vi "MessageReceiver_NewParse.vi"(0 "STOMP In":refnum<class "STOMP.lvclass">, 5 "error in (no error)":errorcluster) -> (14 "STOMP out":refnum<class "STOMP.lvclass">, 19 "error out":errorcluster)   [LabVIEW 2017, in "LabVIEW STOMP.lvlib" / "STOMP.lvclass"]
uses:
  STOMP.lvclass
  Typedefs/Type_MessageParserState.ctl
  Typedefs/Type_ServerFrame.ctl
  Typedefs/Type_ServerFrameType.ctl
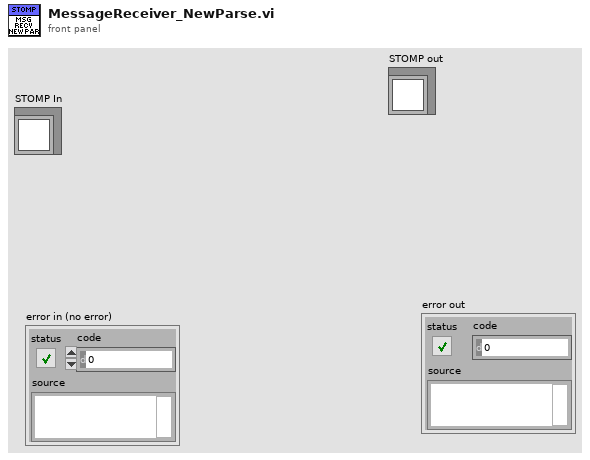
[diagram p1: front panel]
types:
  T1 = typedef "LabVIEW STOMP.lvlib/STOMP.lvclass/Type_ServerFrame.ctl" = cluster{"Type":T2, "Headers":cluster{"Header":string, "Value":string}[], "Body":string}
  T2 = typedef "LabVIEW STOMP.lvlib/STOMP.lvclass/Type_ServerFrameType.ctl" = enum16{"Undefined", "MESSAGE", "CONNECTED", "RECEIPT", "ERROR"}
  T3 = typedef "LabVIEW STOMP.lvlib/STOMP.lvclass/Type_MessageParserState.ctl" = enum16{"WaitForFrame", "ReadCommand", "ReadHeaders", "ReadBody", "FrameReady"}
  T4 = enum16{"Standard", "Buffered", "CRLF", "Immediate"}
  T5 = typedef "STOMP Connection Manager.lvclass/ObjectAttributes.ctl" = cluster{"address":string, "port":u16, "ConnectionRef":refnum<k5>, "messageQueue":refnum<queue>, "receiptQueue":refnum<queue>, "errorQueue":refnum<queue>, "sendQueue":refnum<queue>, "currentReceiptNumber":u64, "currentSubscriptionId":u64, "closeConnection":bool, "activeSubscriptions":T6[]}
  T6 = typedef "LabVIEW STOMP.lvlib/STOMP.lvclass/Type_ActiveSubscription.ctl" = cluster{"id":u64, "receipt":bool, "Destination":string, "ack":T7, "headers":T8[]}
  T7 = typedef "LabVIEW STOMP.lvlib/STOMP.lvclass/Type_AckHeader.ctl" = enum16{"auto", "client", "client-individual"}
  T8 = typedef "LabVIEW STOMP.lvlib/STOMP.lvclass/Type_FrameHeader.ctl" = cluster{"Header":string, "Value":string}
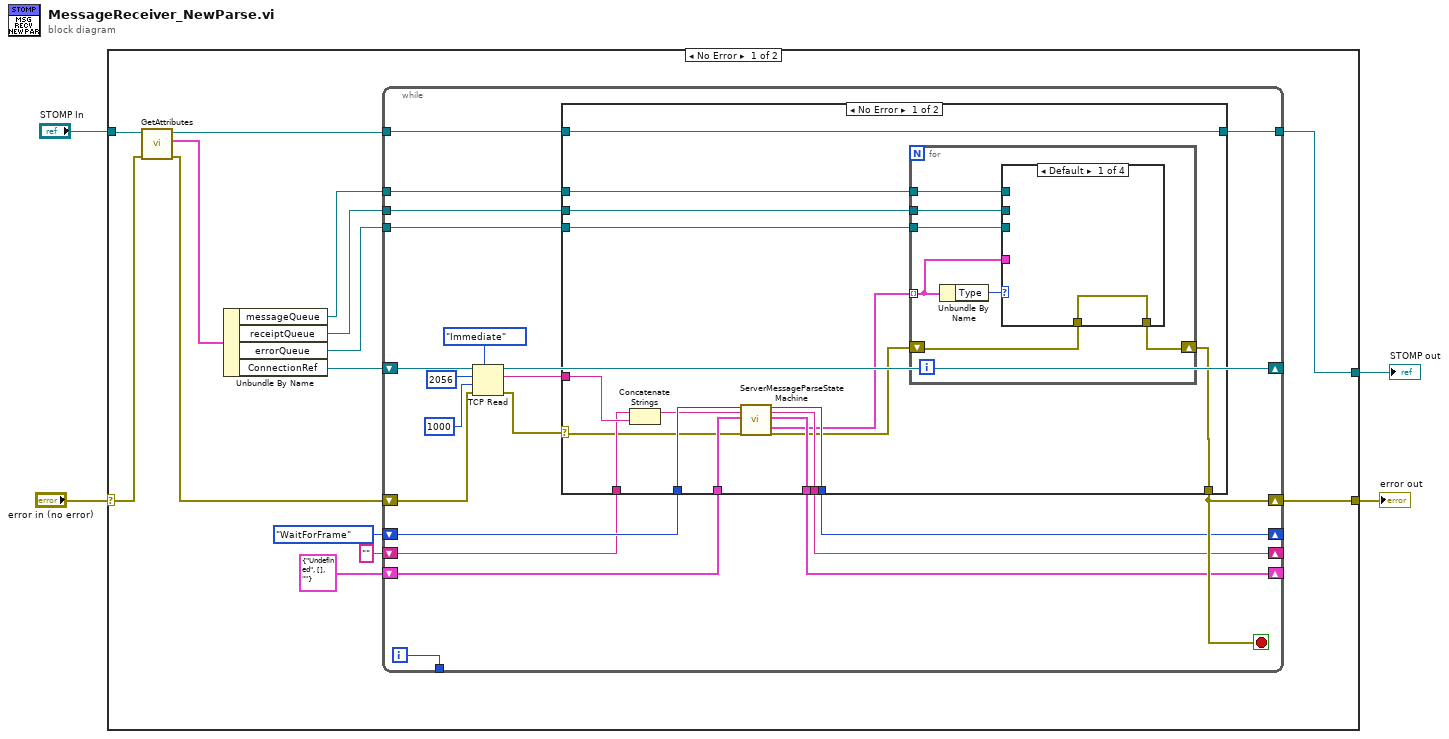
[diagram p0: block diagram]
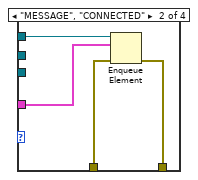
[diagram p2: hidden frame]
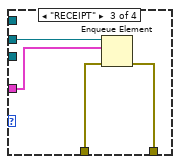
[diagram p3: hidden frame]
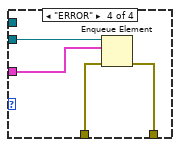
[diagram p4: hidden frame]
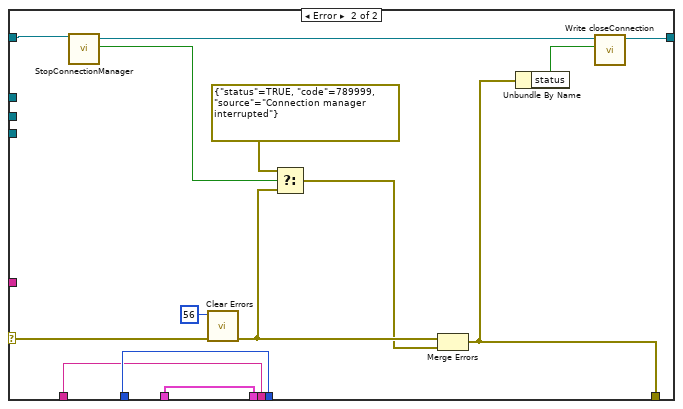
[diagram p5: hidden frame]
diagram:
  n1 = case shown="No Error" "error in (no error)" {
    selector: "error in (no error)" -> [w10 w91]
    tunnel: [w14 w91] -> w4
    tunnel: "STOMP In" -> [w12 w90]
    tunnel: [w13 w90] -> w2
    frame No Error {
      n2 = call-dynamic "GetAttributes.vi"("error in (no error)"=w10, "STOMP in"=w12) -> ("error out"=w9:errorcluster, "attributes"=w8:T5, "STOMP out"=w11:refnum<class "STOMP.lvclass">)  [unwired: 7 in]
      n3 = Unbundle By Name(w8) -> ("messageQueue"=w17:refnum<queue>, "receiptQueue"=w16:refnum<queue>, "errorQueue"=w15:refnum<queue>, "ConnectionRef"=w18:refnum<k5>)
      n4 = while {
        shift-right: [w36] -> _
        shift-left: w18 -> [w37]
        tunnel: w17 -> [w35]
        tunnel: w16 -> [w32]
        tunnel: w15 -> [w31]
        tunnel: [w30] -> _
        shift-right: [w29] -> w14
        shift-left: w9 -> [w34]
        tunnel: w11 -> [w27]
        tunnel: [w26] -> w13
        shift-right: [w24] -> _
        shift-left: Type_MessageParserState."WaitForFrame" ("CurrentState") -> [w21]
        shift-right: [w23] -> _
        shift-left: "" ("CurrentDataBuffer") -> [w20]
        shift-right: [w22] -> _
        shift-left: T1 {"Type"=enum."Undefined", "Headers"=[], "Body"=""} ("CurrentFrameState") -> [w19]
        i -> [w30]
        stop <- w29 stop-if-true
        n5 = TCP Read(connection ID=w37, bytes to read=2056, error in (no error)=w34, 7:T4."Immediate" ("mode (standard)"), 9:1000 ("timeout ms (25000)")) -> (connection ID out=w36:refnum<k5>, data out=w25:string, error out=w28:errorcluster)
        n6 = case shown="No Error" w28 {
          selector: w28 -> [w42 w88]
          tunnel: w25 -> [w46 _]
          tunnel: w35 -> [w55 _]
          tunnel: w32 -> [w54 _]
          tunnel: w31 -> [w53 _]
          tunnel: [w52 w79] -> w29
          tunnel: w27 -> [w51 w87]
          tunnel: [w51 w81] -> w26
          tunnel: [w50 w78] -> w24
          tunnel: [w49 w76] -> w23
          tunnel: [w48 w77] -> w22
          tunnel: w21 -> [w47 w78]
          tunnel: w20 -> [w44 w76]
          tunnel: w19 -> [w43 w77]
          frame No Error {
            n7 = Concatenate Strings(w44, w46) -> (w45:string)
            n8 = call "ServerMessageParseStateMachine.vi"("LastState"=w47, "LastDataBuffer"=w45, "LastFrameState"=w43, "error in"=w42) -> ("CurrentState"=w50:T3, "CurrentDataBuffer"=w49:string, "CurrentFrameState"=w48:T1, "ReadyFrames"=w40:T1[], "error out"=w41:errorcluster)  [unwired: 11 in]
            n9 = for {
              tunnel: w55 -> [w62]
              tunnel: w54 -> [w61]
              tunnel: w53 -> [w60]
              shift-right: [w59] -> w52
              shift-left: w41 -> [w57]
              tunnel: w40 -> [w56] mode=indexing
              n10 = Unbundle By Name(w56) -> ("Type"=w58:T2)
              n11 = case shown="Default" w58 {
                tunnel: w62 -> [_ w67 _ _]
                tunnel: [w63 w66 w71 w75] -> w59
                tunnel: w57 -> [w63 w65 w70 w74]
                tunnel: w61 -> [_ _ w69 _]
                tunnel: w60 -> [_ _ _ w73]
                tunnel: w56 -> [_ w64 w68 w72]
                frame Default {
                }
                frame "MESSAGE", "CONNECTED" {
                  n12 = Enqueue Element(queue=w67, element=w64, error in (no error)=w65) -> (error out=w66:errorcluster)  [unwired: 1 in, 2 out]
                }
                frame "RECEIPT" {
                  n13 = Enqueue Element(queue=w69, element=w68, error in (no error)=w70) -> (error out=w71:errorcluster)  [unwired: 1 in, 2 out]
                }
                frame "ERROR" {
                  n14 = Enqueue Element(queue=w73, element=w72, error in (no error)=w74) -> (error out=w75:errorcluster)  [unwired: 1 in, 2 out]
                }
              }
            }
          }
          frame Error {
            n15 = call-dynamic "StopConnectionManager.vi"("STOMP in"=w87) -> ("STOMP out"=w82:refnum<class "STOMP.lvclass">, "stop?"=w86:bool)  [unwired: 16 in, 1 out]
            n16 = call <vilib>:"Clear Errors.vi"("error in (no error)"=w88, "specific error code to clear (0: all)"=56) -> ("error out"=w84:errorcluster)  [unwired: 4 in, 1 out]
            n17 = Select(t=errorcluster {"status"=TRUE, "code"=789999, "source"="Connection manager interrupted"} ("error constant"), s=w86, f=w84) -> (s? t:f=w83:errorcluster)
            n18 = Merge Errors(w84, w83) -> (w79:errorcluster)
            n19 = Unbundle By Name(w79) -> ("status"=w80:bool)
            n20 = call-dynamic "Write closeConnection.vi"("closeConnection"=w80, "STOMP in"=w82) -> ("STOMP out"=w81:refnum<class "STOMP.lvclass">)  [unwired: 8 in, 1 out]
          }
        }
      }
    }
    frame Error {
    }
  }
  "error out" <- w4
  "STOMP out" <- w2
